vi "探头窗口-32-4列-网络版.vi"() -> ()   [LabVIEW 2017]
panel:
  in  "外部停止命令？":bool=TRUE
  out "引用-监测模式？":refnum<vi>
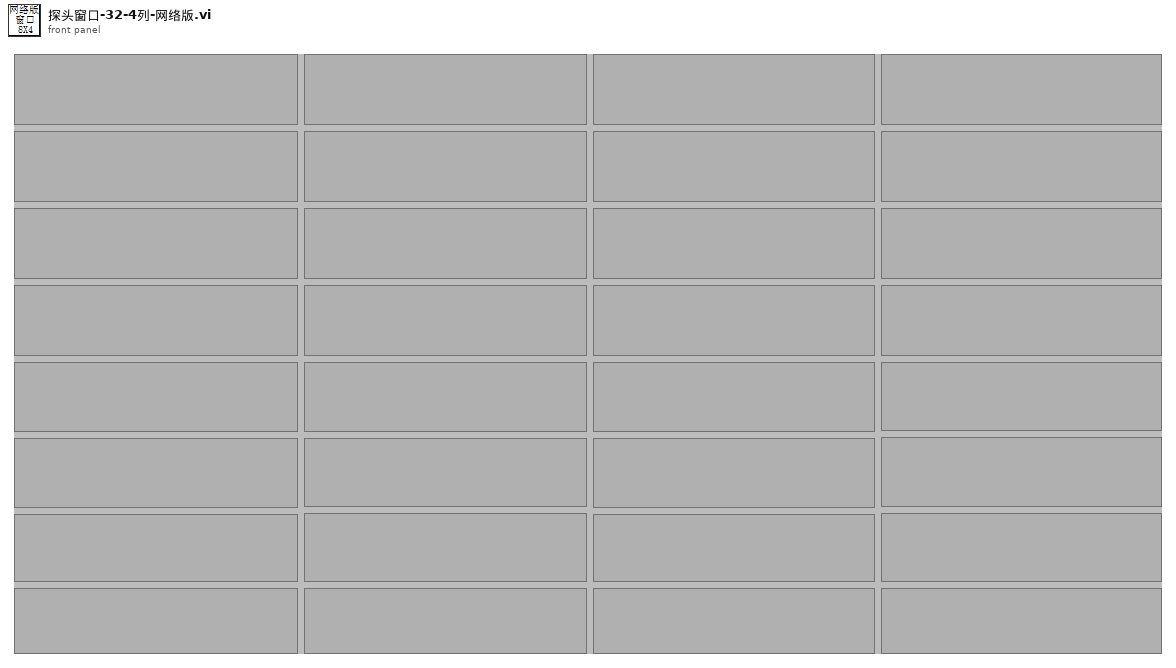
[diagram p1: front panel]
types:
  T1 = typedef "eventvkey.ctl" = enum16{"ASCII", "Enter", "Return", "Shift", "Ctrl", "Alt", "Cmd", "Opt", "Caps", "NumLock", "Clear", "Break", "Up", "Down", "Left", "Right", "Insert", "Delete", "Home", "End", "PageUp", "PageDown", "Escape", "Help", "Pause", "ScrollLock", "F1", "F2", "F3", "F4", "F5", "F6", "F7", "F8", "F9", "F10", "F11", "F12", "F13", "F14", "F15", "F16", "F17", "F18", "F19", "F20", "F21", "F22", "F23", "F24", "Play", "VolumeUp", "VolumeDown", "Mute", "Two Byte Char"}
  T2 = typedef "探头属性.ctl" = cluster{"探头地址与信息":T3, "测量值":T6, "限值":T7, "探头状态":T8, "累积记录":T9, "报警方式":T10}
  T3 = typedef "探测器信息.ctl" = cluster{"网络地址":string, "名称":string, "备注":string, "累积剂量":dbl, "累积限值":dbl, "硬件剂量率限值":T4, "剂量率限值1":dbl, "剂量率限值2":dbl, "报警方式":T5}
  T4 = typedef "探头剂量率限值选择.ctl" = enum16{"一级限值", "二级限值"}
  T5 = typedef "报警方式选择.ctl" = enum16{"常报警", "自动静音", "手动静音"}
  T6 = typedef "测量值.ctl" = cluster{"时间":timestamp, "数值":dbl}
  T7 = typedef "剂量率限值.ctl" = cluster{"限值1":dbl, "限值2":dbl, "探头限值":T4}
  T8 = typedef "探头状态.ctl" = enum16{"正常", "离线", "禁用", "一级报警", "二级报警", "累积报警"}
  T9 = typedef "单条累积记录.ctl" = cluster{"起始时间":timestamp, "结束时间":timestamp, "累积剂量":dbl}
  T10 = typedef "报警方式.ctl" = cluster{"报警方式":T5, "延迟计时":u16, "报警中？":bool}
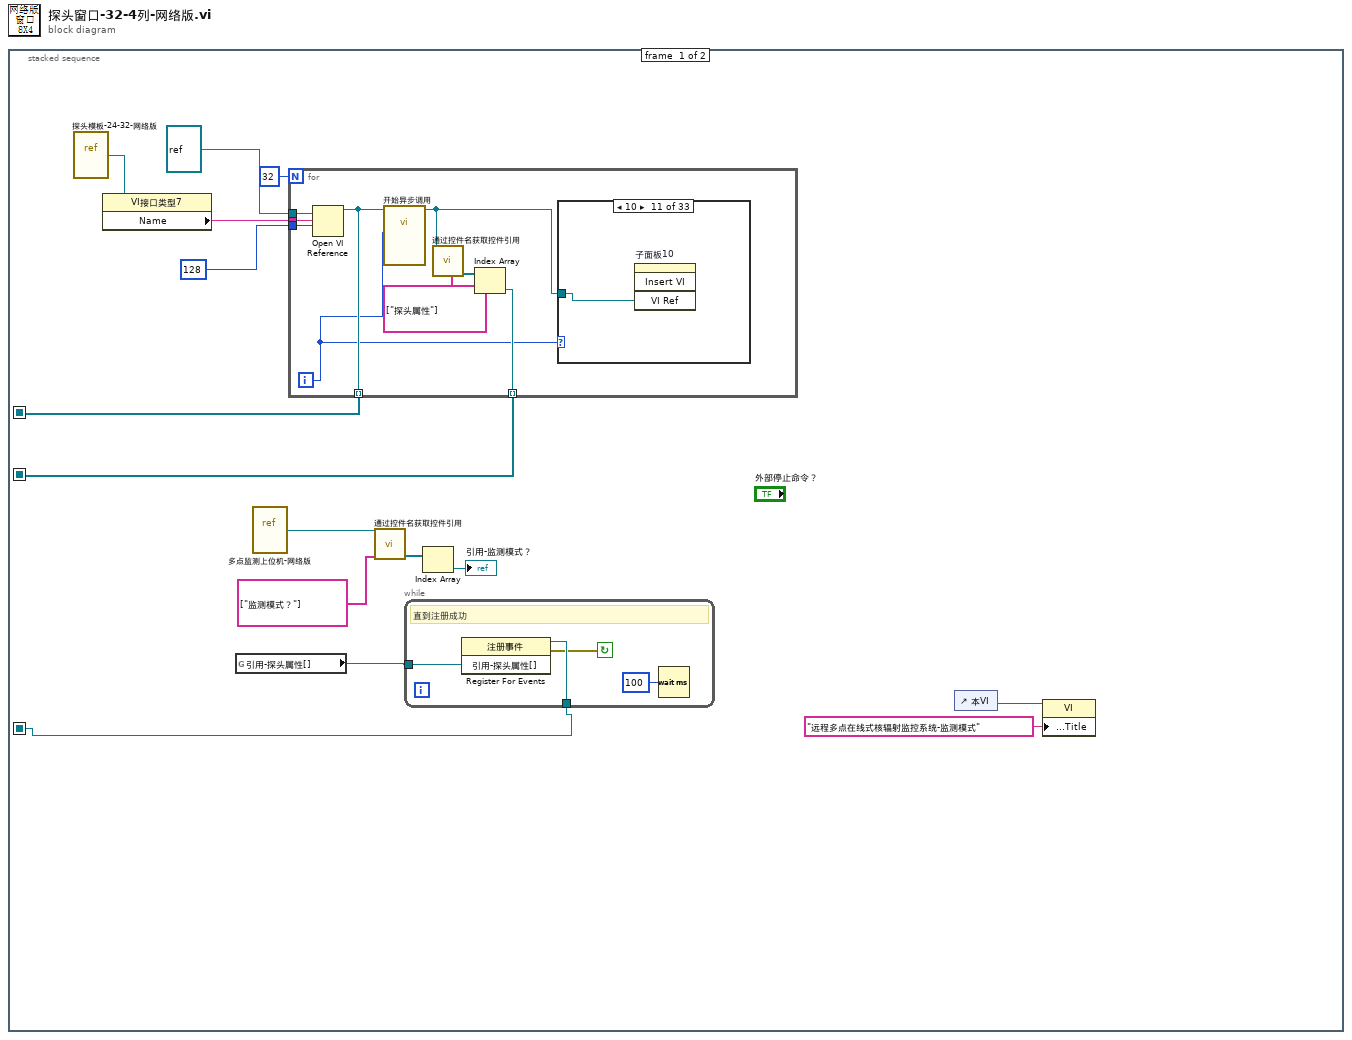
[diagram p0: block diagram]
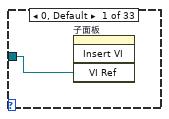
[diagram p2: hidden frame]
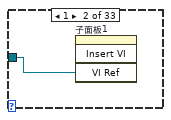
[diagram p3: hidden frame]
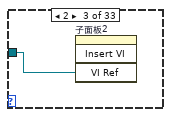
[diagram p4: hidden frame]
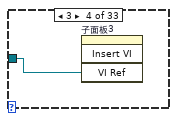
[diagram p5: hidden frame]
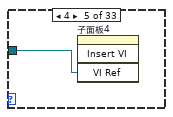
[diagram p6: hidden frame]
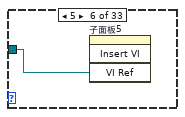
[diagram p7: hidden frame]
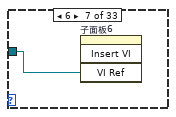
[diagram p8: hidden frame]
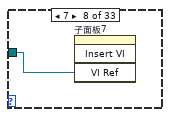
[diagram p9: hidden frame]
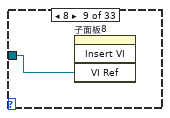
[diagram p10: hidden frame]
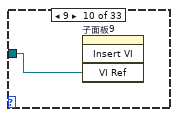
[diagram p11: hidden frame]
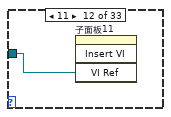
[diagram p12: hidden frame]
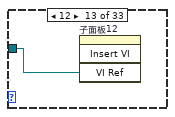
[diagram p13: hidden frame]
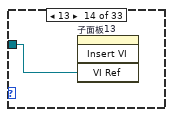
[diagram p14: hidden frame]
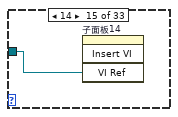
[diagram p15: hidden frame]
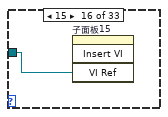
[diagram p16: hidden frame]
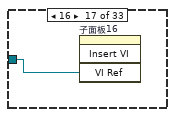
[diagram p17: hidden frame]
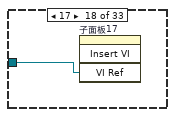
[diagram p18: hidden frame]
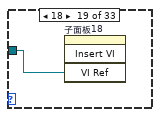
[diagram p19: hidden frame]
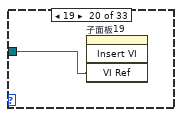
[diagram p20: hidden frame]
diagram:
  n1 = stacked-sequence {
    seq-local: [w10 _] -> [_ w63]
    seq-local: [w9 _] -> [_ w62]
    seq-local: [w1 _] -> [_ w61]
    frame #0 {
      n2 = vi-ref "探头模板-24-32-网络版.vi"() -> (w15:refnum<vi>)
      n3 = property class="VI接口类型7"(reference=w15) -> ("Name"=w14:string)  [unwired: 1 in, 2 out]
      n4 = global read "全局变量-35点监测.vi" "引用-探头属性[]"() -> (w2:refnum<vi>)
      n5 = vi-ref "多点监测上位机-网络版.vi"() -> (w8:refnum<vi>)
      n6 = for {
        N: 32 -> [_]
        tunnel: w14 -> [w28]
        tunnel: 128 ("选项") -> [w27]
        tunnel: refnum<vi> refnum ("类型说明符VI引用句柄（仅用于类型）") -> [w26]
        tunnel: [w22] -> w10 mode=indexing
        tunnel: [w23] -> w9 mode=indexing
        i -> [w20]
        n7 = Open VI Reference(type specifier VI Refnum (for type only)=w26, vi path=w28, options=w27) -> (vi reference=w22:refnum<vi>)  [unwired: 3 in, 1 out]
        n8 = call-by-ref "开始异步调用"(reference=w22, "探头序号"=w20) -> (reference out=w21:refnum<vi>)  [unwired: 12 in, 1 out]
        n9 = call "通过控件名获取控件引用.vi"("控件名数组"=string[] ["探头属性"], "VI引用"=w21) -> ("控件引用输出"=w24:refnum<vi>[])  [unwired: 7 in, 2 out]
        n10 = Index Array(array=w24) -> (element=w23:refnum<vi>)  [unwired: 1 in]
        n11 = case shown="10" w20 {
          tunnel: w21 -> [w29 w30 w31 w32 w33 w34 w35 w36 w37 w38 w39 w40 w41 w42 w43 w44 w45 w46 w47 w48 w49 w50 w51 w52 w53 w54 w55 w56 w57 w58 w59 w60 _]
          frame 0, Default {
            n12 = invoke on="子面板" class="子面板" method="Insert VI"("VI Ref"=w29) -> ()  [unwired: 3 in, 4 out]
          }
          frame 1 {
            n13 = invoke on="子面板1" class="SubPnl" method="Insert VI"("VI Ref"=w30) -> ()  [unwired: 3 in, 4 out]
          }
          frame 2 {
            n14 = invoke on="子面板2" class="SubPnl" method="Insert VI"("VI Ref"=w31) -> ()  [unwired: 3 in, 4 out]
          }
          frame 3 {
            n15 = invoke on="子面板3" class="SubPnl" method="Insert VI"("VI Ref"=w32) -> ()  [unwired: 3 in, 4 out]
          }
          frame 4 {
            n16 = invoke on="子面板4" class="SubPnl" method="Insert VI"("VI Ref"=w33) -> ()  [unwired: 3 in, 4 out]
          }
          frame 5 {
            n17 = invoke on="子面板5" class="SubPnl" method="Insert VI"("VI Ref"=w34) -> ()  [unwired: 3 in, 4 out]
          }
          frame 6 {
            n18 = invoke on="子面板6" class="SubPnl" method="Insert VI"("VI Ref"=w35) -> ()  [unwired: 3 in, 4 out]
          }
          frame 7 {
            n19 = invoke on="子面板7" class="SubPnl" method="Insert VI"("VI Ref"=w36) -> ()  [unwired: 3 in, 4 out]
          }
          frame 8 {
            n20 = invoke on="子面板8" class="SubPnl" method="Insert VI"("VI Ref"=w37) -> ()  [unwired: 3 in, 4 out]
          }
          frame 9 {
            n21 = invoke on="子面板9" class="SubPnl" method="Insert VI"("VI Ref"=w38) -> ()  [unwired: 3 in, 4 out]
          }
          frame 10 {
            n22 = invoke on="子面板10" class="SubPnl" method="Insert VI"("VI Ref"=w39) -> ()  [unwired: 3 in, 4 out]
          }
          frame 11 {
            n23 = invoke on="子面板11" class="SubPnl" method="Insert VI"("VI Ref"=w40) -> ()  [unwired: 3 in, 4 out]
          }
          frame 12 {
            n24 = invoke on="子面板12" class="SubPnl" method="Insert VI"("VI Ref"=w41) -> ()  [unwired: 3 in, 4 out]
          }
          frame 13 {
            n25 = invoke on="子面板13" class="SubPnl" method="Insert VI"("VI Ref"=w42) -> ()  [unwired: 3 in, 4 out]
          }
          frame 14 {
            n26 = invoke on="子面板14" class="SubPnl" method="Insert VI"("VI Ref"=w43) -> ()  [unwired: 3 in, 4 out]
          }
          frame 15 {
            n27 = invoke on="子面板15" class="SubPnl" method="Insert VI"("VI Ref"=w44) -> ()  [unwired: 3 in, 4 out]
          }
          frame 16 {
            n28 = invoke on="子面板16" class="SubPnl" method="Insert VI"("VI Ref"=w45) -> ()  [unwired: 3 in, 4 out]
          }
          frame 17 {
            n29 = invoke on="子面板17" class="SubPnl" method="Insert VI"("VI Ref"=w46) -> ()  [unwired: 3 in, 4 out]
          }
          frame 18 {
            n30 = invoke on="子面板18" class="SubPnl" method="Insert VI"("VI Ref"=w47) -> ()  [unwired: 3 in, 4 out]
          }
          frame 19 {
            n31 = invoke on="子面板19" class="SubPnl" method="Insert VI"("VI Ref"=w48) -> ()  [unwired: 3 in, 4 out]
          }
          frame 20 {
            n32 = invoke on="子面板20" class="SubPnl" method="Insert VI"("VI Ref"=w49) -> ()  [unwired: 3 in, 4 out]
          }
          frame 21 {
            n33 = invoke on="子面板21" class="SubPnl" method="Insert VI"("VI Ref"=w50) -> ()  [unwired: 3 in, 4 out]
          }
          frame 22 {
            n34 = invoke on="子面板22" class="SubPnl" method="Insert VI"("VI Ref"=w51) -> ()  [unwired: 3 in, 4 out]
          }
          frame 23 {
            n35 = invoke on="子面板23" class="SubPnl" method="Insert VI"("VI Ref"=w52) -> ()  [unwired: 3 in, 4 out]
          }
          frame 24 {
            n36 = invoke on="子面板24" class="SubPnl" method="Insert VI"("VI Ref"=w53) -> ()  [unwired: 3 in, 4 out]
          }
          frame 25 {
            n37 = invoke on="子面板25" class="SubPnl" method="Insert VI"("VI Ref"=w54) -> ()  [unwired: 3 in, 4 out]
          }
          frame 26 {
            n38 = invoke on="子面板26" class="SubPnl" method="Insert VI"("VI Ref"=w55) -> ()  [unwired: 3 in, 4 out]
          }
          frame 27 {
            n39 = invoke on="子面板27" class="SubPnl" method="Insert VI"("VI Ref"=w56) -> ()  [unwired: 3 in, 4 out]
          }
          frame 28 {
            n40 = invoke on="子面板28" class="SubPnl" method="Insert VI"("VI Ref"=w57) -> ()  [unwired: 3 in, 4 out]
          }
          frame 29 {
            n41 = invoke on="子面板29" class="SubPnl" method="Insert VI"("VI Ref"=w58) -> ()  [unwired: 3 in, 4 out]
          }
          frame 30 {
            n42 = invoke on="子面板30" class="SubPnl" method="Insert VI"("VI Ref"=w59) -> ()  [unwired: 3 in, 4 out]
          }
          frame 31 {
            n43 = invoke on="子面板31" class="SubPnl" method="Insert VI"("VI Ref"=w60) -> ()  [unwired: 3 in, 4 out]
          }
          frame 32 {
          }
        }
      }
      n44 = call "通过控件名获取控件引用.vi"("控件名数组"=string[] ["监测模式？"], "VI引用"=w8) -> ("控件引用输出"=w6:refnum<vi>[])  [unwired: 7 in, 2 out]
      n45 = while {
        tunnel: w2 -> [w19]
        tunnel: [w18] -> w1
        stop <- w17 continue-if-true
        # "直到注册成功"
        n46 = register-events(w19) -> (reference out=w18:refnum<event-registration>, error out=w17:errorcluster)  [unwired: 2 in]
        n47 = Wait (ms)(milliseconds to wait=u32 100 ("等待时间（毫秒）")) -> ()  [unwired: 1 out]
      }
      n48 = Index Array(array=w6) -> (element=→"引用-监测模式？":refnum<vi>)  [unwired: 1 in]
      n49 = control-ref of="本VI"() -> (w4:refnum<vi>)
      n50 = property class="VI"(reference=w4, "Front Panel.Title"="远程多点在线式核辐射监控系统-监测模式" ("前面板窗口:标题")) -> ()  [unwired: 1 in, 2 out]
    }
    frame #1 {
      n51 = while {
        tunnel: w63 -> [w66]
        tunnel: w62 -> [w65]
        tunnel: w61 -> [w64]
        stop <- w67 stop-if-true
        n52 = event shown="[3] \"外部停止命令？\": 值改变" {
          selector: w64 -> [_ _ _ w72 _]
          dyn-events: _ -> [_ _ _ _ _]
          timeout: _ -> [_ _ _ _ _]
          tunnel: [_ _ _ TRUE ("放弃？") _] -> w67
          tunnel: w66 -> [_ _ _ w74 _]
          tunnel: w65 -> [_ _ _ _ w90]
          event Timeout {
            n53 = event-data() -> ()  [unwired: 1 in, 3 out]
          }
          event Panel Close? {
            n54 = event-data() -> ()  [unwired: 1 in, 4 out]
            n55 = property on="外部停止命令？" class="Bool (严格)"("Val(Sgnl)"=FALSE ("值(信号)")) -> ()  [unwired: 2 in, 2 out]
            n56 = event-data("Discard?"=TRUE ("放弃？")) -> ()  [unwired: 1 in, 1 out]
          }
          event Key Down {
            n57 = event-data() -> ("VKey"=w70:T1)  [unwired: 1 in, 9 out]
            n58 = case shown="\"Enter\"" w70 {
              frame "ASCII", Default {
              }
              frame "Enter" {
                # "退出"
                n59 = property on="外部停止命令？" class="Bool (严格)"("Val(Sgnl)"=FALSE ("值(信号)")) -> ()  [unwired: 2 in, 2 out]
              }
            }
          }
          event "外部停止命令？": Value Change {
            # "注销事件，防止“探头属性值改变”事件自动触发 ，导致前面板锁定"
            n60 = event-data() -> ()  [unwired: 1 in, 6 out]
            n61 = flat-sequence {
              tunnel: w74 -> [w77]
              tunnel: [w77] -> w73
              tunnel: w72 -> [w76]
              tunnel: w73 -> [w84]
              frame #0 {
                n62 = Unregister For Events(event registration refnum=w76) -> ()  [unwired: 1 in, 1 out]
              }
              frame #1 {
                w83 = FALSE  # F
                n63 = for {
                  tunnel: w84 -> [w89] mode=indexing
                  tunnel: [w85] -> w80
                  n64 = invoke class="VI (严格)" method="Abort VI"(reference=w89) -> (reference out=w87:refnum<vi>, error out=w88:errorcluster)  [unwired: 2 in, 1 out]
                  n65 = Close Reference(reference=w87, error in (no error)=w88) -> (error out=w86:errorcluster)
                  n66 = call <vilib>:"Clear Errors.vi"("error in (no error)"=w86) -> ("error out"=w85:errorcluster)  [unwired: 5 in, 1 out]
                }
                n67 = local read "引用-监测模式？"() -> (w82:refnum<vi>)
                n68 = control-ref of="本VI"() -> (w81:refnum<vi>)
                n69 = property class="Ctl"(reference=w82, error in=w80, "Val(Sgnl)"=w83) -> (error out=w79:errorcluster)  [unwired: 1 out]
                n70 = invoke class="VI" method="FP.Close"(reference=w81, error in=w79) -> (error out=w78:errorcluster)  [unwired: 1 in, 2 out]
                n71 = call <vilib>:"Clear Errors.vi"("error in (no error)"=w78) -> ()  [unwired: 5 in, 2 out]
              }
            }
          }
          event Value Change {
            n72 = event-data() -> ("NewVal"=w91:T2[])  [unwired: 1 in, 5 out]
            n73 = for {
              workers-P: _ -> [_]
              tunnel: w90 -> [w93] mode=indexing
              tunnel: w91 -> [w92] mode=indexing
              # "各个“探头属性”赋值（信号）"
              n74 = property class="Ctl"(reference=w93, "Val(Sgnl)"=w92) -> ()  [unwired: 1 in, 2 out]
            }
          }
        }
      }
    }
  }
